vi "Global Controls.vi"() -> ()   [LabVIEW 2020]
uses:
  _Controls/Confocal Controls.ctl
  _Controls/MCSL Controls.ctl
  _Controls/Spots.ctl
  _Controls/SLM Real World to IMAQ Display Transform.ctl
  _Controls/iFlex.ctl
  _Controls/Tweezertron Ctrl Refs.ctl
  _Controls/PIFOC Position.ctl
  _Controls/Manlight Controls.ctl
  _Controls/Exp Params.ctl
  _Controls/Image Thresholds.ctl
  _Controls/Review Ctrl Refs.ctl
panel:
  in  "Review Ctrl Refs":T1
  in  "Stop Experiment":bool
  in  "Exp Params":T2={"Experiment Type"="2D Snapshot", "Experiment Name"="Experiment_1", "ExpPath"=path "E:/Data", "TSFrames"=1000, "TSfps"=1000, "ZTSFrames"=1000, "ZTSdt"=1, "Streaming"=FALSE, "Z Stack Settings"={"Start"=0.0, "Step Size"=0.1, "Finish"=1.0}, "total images"=1, "tdms ref"=refnum, "frame #"=0, "images per stack"=1, "total stacks"=1, "period"=1, "PI MVR Increment"=""} {"period" min=1; "total stacks" min=1; "images per stack" min=1; "total images" min=1; "Z Stack Settings"."Start" min=0.0 max=100.0 step=0.1; "Z Stack Settings"."Step Size" min=0.1 max=100.0 step=0.1; "Z Stack Settings"."Finish" min=0.0 max=100.0 step=0.1; "TSFrames" min=1 step=1; "ZTSdt" min=1 step=1; "ZTSFrames" min=2 step=1; "TSfps" min=1 max=1000 step=1}
  in  "PinSelector":dbl(ring)=6.0 caption="Pin Hole" items=["25", "30", "35", "40", "45", "50", "60", "70", "80", "90", "100", "125", "200", "300", "1000", "2000"]
  in  "PIFOC Settings":T3 {"PIFOC Position\n(um) [ACT]" format="%.2f"; "PIFOC Position (mm) [SET]" min=0.0 max=100.0 step=0.1 scale=0.0..100.0}
  out "Tweezertron Ctrl Refs":T4
  in  "iFlex Controls":T5 {"561" min=12.5 max=100.0 step=0.1 scale=0.0..100.0; "488" min=30.0 max=100.0 step=0.1 scale=0.0..100.0}
  in  "SLM to IMAQ":T6={"Translation"={"X"=255.9856, "Y"=245.976}, "Scalling"={"xScale"=2.61758691206544, "yScale"=-2.61759}}
  in  "Spots":T7={"Spot Params"=[{"Intensity"=1.0, "Vortex"=0.0, "Phase"=0.0, "X"=0.0, "Y"=0.0, "Z"=0.0}, {"Intensity"=0.0, "Vortex"=0.0, "Phase"=0.0, "X"=0.0, "Y"=0.0, "Z"=0.0}], "Add Spot"=FALSE, "Remove Spot"=FALSE, "Clear All Spots"=FALSE, "Save Spots"=FALSE, "Generate Spots"=FALSE, "Generate Spot Pattern"=""} {"Spot Params"."Z" format="%_4g"; "Spot Params"."Y" format="%_4g"; "Spot Params"."X" format="%_4g"; "Spot Params"."Phase" format="%_4g"; "Spot Params"."Intensity" format="%_4g"}
  in  "MCSL Controls":T8={"405"={"Enable"=FALSE, "Power (%)"=0.0}, "488"={"Enable"=FALSE, "Power (%)"=55.0}, "642"={"Enable"=FALSE, "Power (%)"=0.0}, "532"={"Enable"=TRUE, "Power (%)"=78.0}} {"532"."Power (%)" min=0.0 max=100.0 step=1.0 scale=0.0..100.0; "642"."Power (%)" min=0.0 max=100.0 step=1.0 scale=0.0..100.0; "488"."Power (%)" min=0.0 max=100.0 step=1.0 scale=0.0..100.0; "405"."Power (%)" min=0.0 max=100.0 step=0.1 scale=0.0..100.0}
  in  "Confocal Controls":T9={"Channel Selection"=enum."AB", "Pixel Count"={"Pixels in X"=512, "Pixels in Y"=512}, "Field Size"=76.0, "Frames"=3, "Averaging"=FALSE, "Alignment"=19.0, "Scan Mode"=TRUE, "Gain"={"Gain A"=25, "Gain B"=5}, "Enable PMTs"={"A"=TRUE, "B"=TRUE}, "Voltage Range"={"Range A"=10, "Range B"=10}, "Multi Frame Count"=0.0, "Trigger Mode"=2.0, "Real Time Averaging"=TRUE, "PFOV"=100.11733333333333, "MicronsPerPx"=0.19554166666667} {"Field Size" min=5.0 max=255.0 step=1.0 scale=5.0..255.0; "PFOV" min=1.0 max=300.0 step=0.1; "MicronsPerPx" min=0.01 step=0.01 format="%.2f"; "Gain"."Gain B" min=1 max=100 step=1; "Gain"."Gain A" min=1 max=100 step=1; "Voltage Range"."Range B" items=["100mV"=5, "200mV"=6, "400mV"=7, "1V"=10, "2V"=11, "4V"=12]; "Voltage Range"."Range A" items=["100mV"=5, "200mV"=6, "400mV"=7, "1V"=10, "2V"=11, "4V"=12]; "Pixel Count"."Pixels in Y" items=["32"=32, "64"=64, "128"=128, "256"=256, "512"=512, "1024"=1024, "2048"=2048]; "Pixel Count"."Pixels in X" items=["32"=32, "64"=64, "128"=128, "256"=256, "512"=512, "1024"=1024, "2048"=2048]}
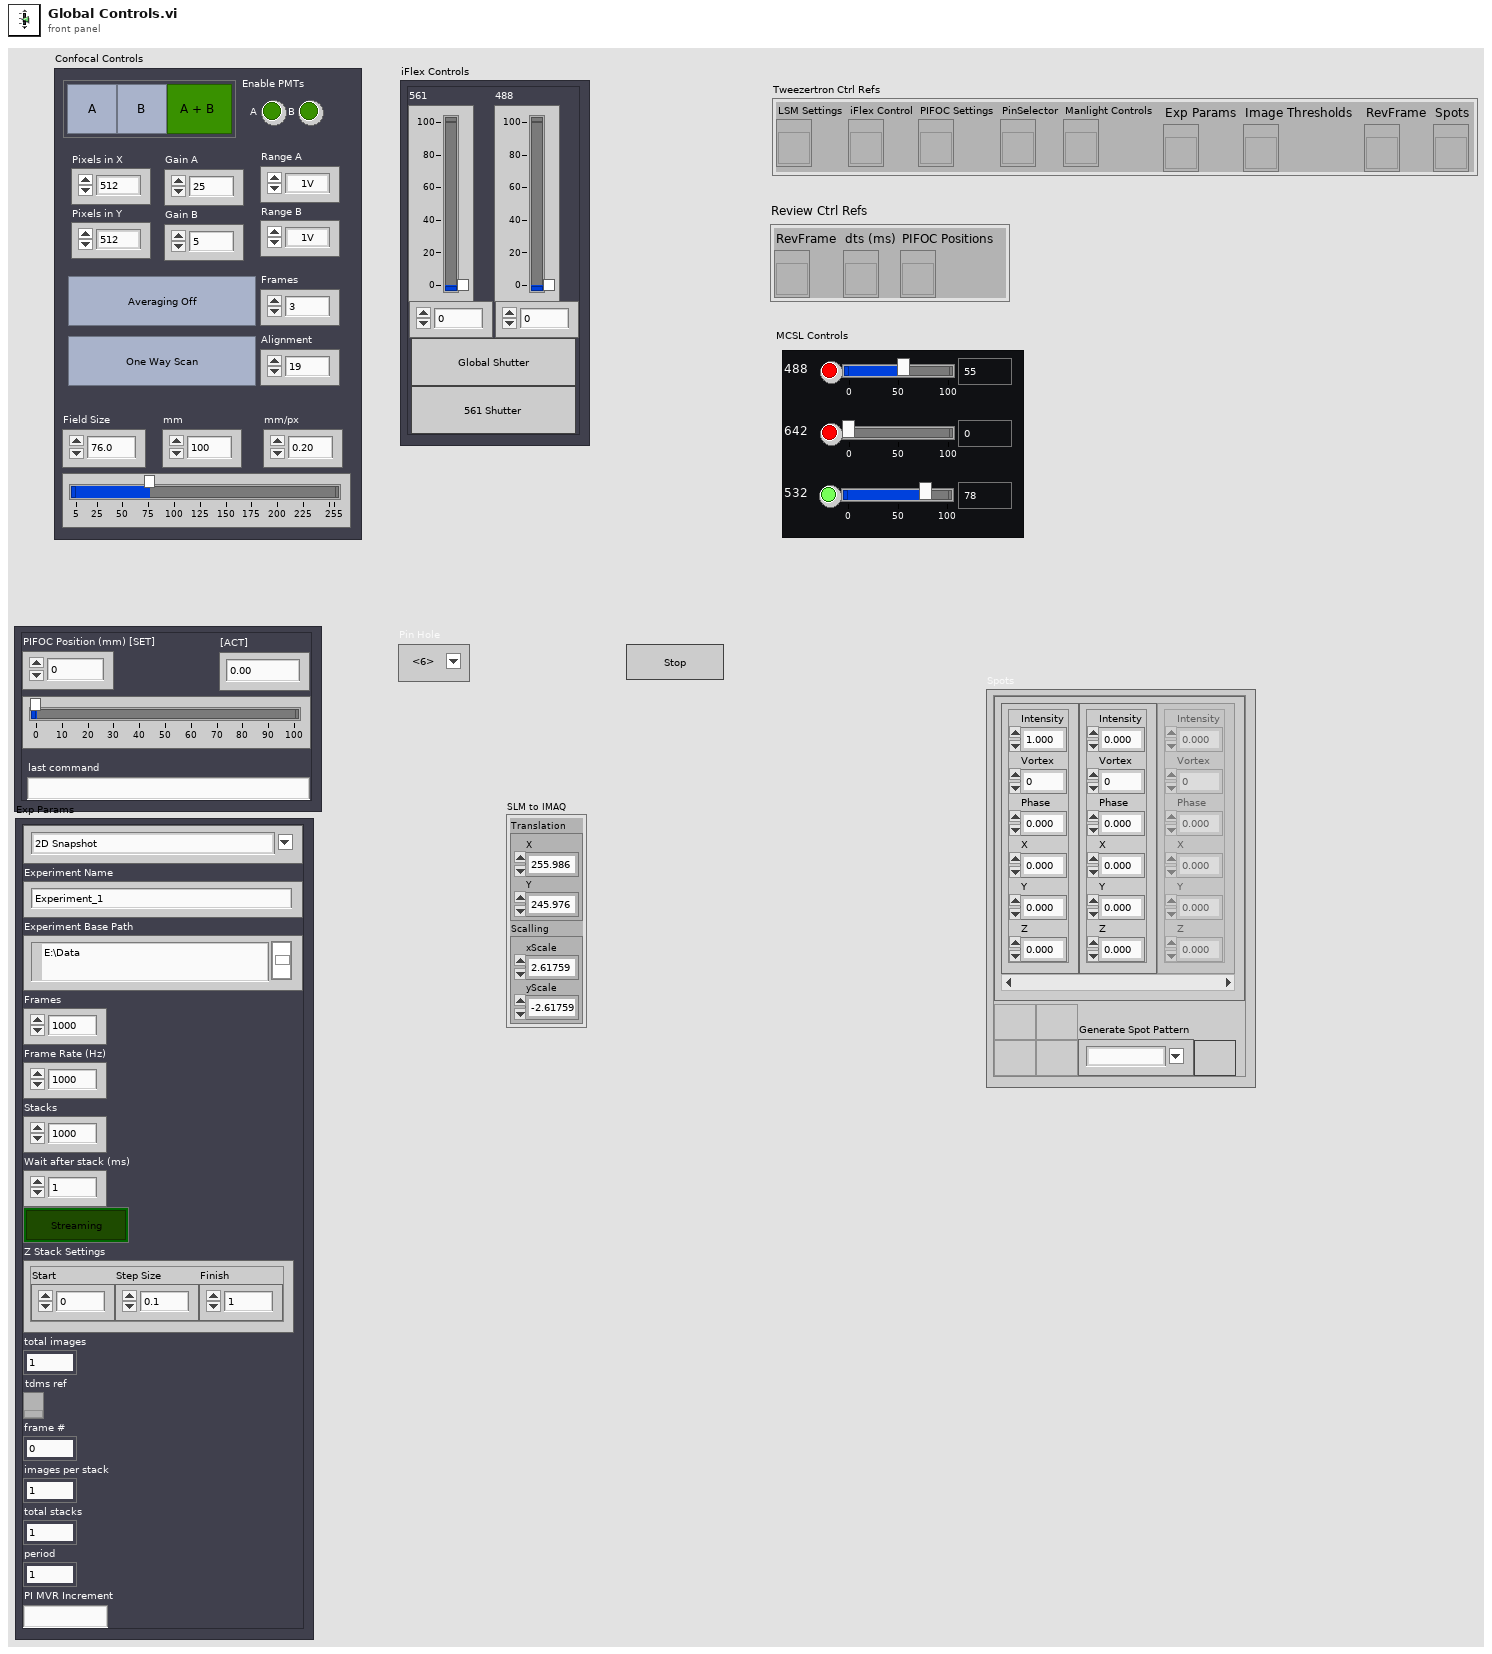
[diagram p1: front panel]
types:
  T1 = typedef "Review Ctrl Refs.ctl" = cluster{"RevFrame":refnum<vi>, "dts (ms)":refnum<vi>, "PIFOC Positions":refnum<vi>}
  T2 = typedef "Exp Params.ctl" = cluster{"Experiment Type":string, "Experiment Name":string, "ExpPath":path, "TSFrames":i32, "TSfps":i32, "ZTSFrames":i32, "ZTSdt":i32, "Streaming":bool, "Z Stack Settings":cluster{"Start":dbl, "Step Size":dbl, "Finish":dbl}, "total images":i32, "tdms ref":refnum<k34>, "frame #":i64, "images per stack":i32, "total stacks":i32, "period":i32, "PI MVR Increment":string}
  T3 = typedef "PIFOC Position.ctl" = cluster{"PIFOC Position (mm) [SET]":dbl, "PIFOC Position\n(um) [ACT]":dbl, "last command":string}
  T4 = typedef "Tweezertron Ctrl Refs.ctl" = cluster{"LSM Settings":refnum<vi>, "iFlex Control":refnum<vi>, "PIFOC Settings":refnum<vi>, "PinSelector":refnum<vi>, "Manlight Controls":refnum<vi>, "Exp Params":refnum<vi>, "Image Thresholds":refnum<vi>, "RevFrame":refnum<vi>, "Spots":refnum<vi>}
  T5 = typedef "iFlex.ctl" = cluster{"561":dbl, "488":dbl, "Global Shutter":bool, "561 Shutter":bool}
  T6 = typedef "SLM Real World to IMAQ Display Transform.ctl" = cluster{"Translation":cluster{"X":dbl, "Y":dbl}, "Scalling":cluster{"xScale":dbl, "yScale":dbl}}
  T7 = typedef "Spots.ctl" = cluster{"Spot Params":cluster{"Intensity":dbl, "Vortex":dbl, "Phase":dbl, "X":dbl, "Y":dbl, "Z":dbl}[], "Add Spot":bool, "Remove Spot":bool, "Clear All Spots":bool, "Save Spots":bool, "Generate Spots":bool, "Generate Spot Pattern":string}
  T8 = typedef "MCSL Controls.ctl" = cluster{"405":cluster{"Enable":bool, "Power (%)":dbl}, "488":cluster{"Enable":bool, "Power (%)":dbl}, "642":cluster{"Enable":bool, "Power (%)":dbl}, "532":cluster{"Enable":bool, "Power (%)":dbl}}
  T9 = typedef "Confocal Controls.ctl" = cluster{"Channel Selection":enum32{"A", "B", "AB"}, "Pixel Count":cluster{"Pixels in X":u32, "Pixels in Y":u32}, "Field Size":dbl, "Frames":u8, "Averaging":bool, "Alignment":dbl, "Scan Mode":bool, "Gain":cluster{"Gain A":u8, "Gain B":u8}, "Enable PMTs":cluster{"A":bool, "B":bool}, "Voltage Range":cluster{"Range A":u16, "Range B":u16}, "Multi Frame Count":dbl, "Trigger Mode":dbl, "Real Time Averaging":bool, "PFOV":dbl, "MicronsPerPx":dbl}
diagram:
